vi "OldUWBController.vi"() -> ()   [LabVIEW 2016]
doc: "The roboRIO Project template acquires acceleration data from the onboard accelerometer and displays the changes of acceleration values in a waveform chart."
uses:
  <vilib>/myRIO/Instrument Drivers/Onboard IO/UART/typedef/VISA Configuration.ctl
  <vilib>/myRIO/Instrument Drivers/Onboard IO/UART/UART.lvlib
  <vilib>/Instr/_visa.llb/VISA Configure Serial Port (Instr).vi
  <vilib>/regexp/Match Regular Expression.xnode
  <vilib>/myRIO/Express VI/Onboard IO/UART/UART Express VI.xnode
panel:
  out "Character Count":u32
  out "UART Reset Buffer":string
  in  "Reset Active\n(Default: ON)":bool
  in  "Delay Time (s)":dbl=10.0
  in  "Stop Program":bool
  out "Z":dbl
  out "Y":dbl
  out "X":dbl
  out "offset past match\n(-1 = no match)":i32
  out "after POS match":string
  out "Characters Read":string
  out "error out OUTPUT":errorcluster
  in  "error in OUTPUT":errorcluster
  out "error out INPUT":errorcluster
  in  "error in INPUT":errorcluster
  # "UART INIT INPUT"
  # "UART OUTPUT"
  # "DEBUG"
  # "COORDINATES"
  # "Input ASCII Codes\n--------------------\nlep - 108, 101, 112\nlec - 108, 101, 99\n\ncr - 13"
  # "STARTUP RESET"
  # "INPUT ERROR"
  # "OUTPUT ERROR"
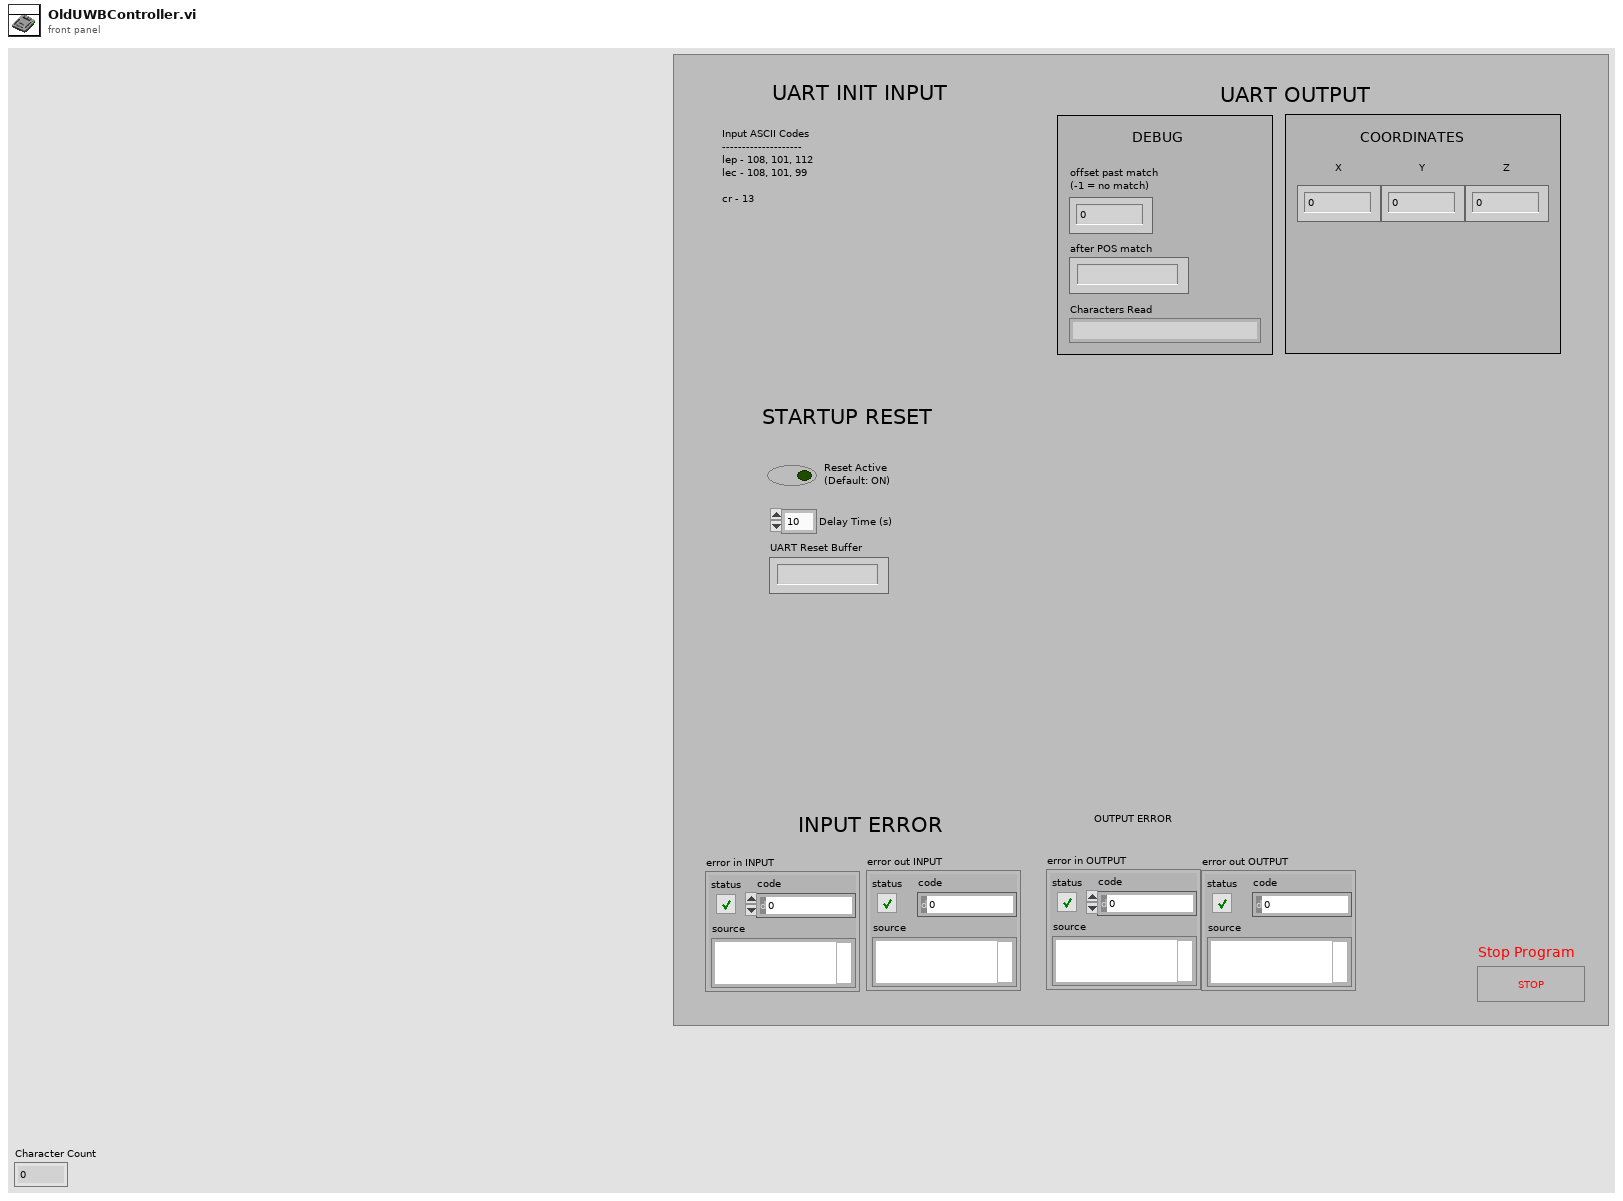
[diagram p1: front panel]
types:
  T1 = typedef "UART.lvlib/VISA Configuration.ctl" = cluster{"baud rate (9600)":u32, "data bits (8)":u16, "parity (0:none)":enum16{"None", "Odd", "Even", "Mark", "Space"}, "stop bits (10: 1 bit)":u16, "flow control (0:none)":u16, "termination char\n(0xA = '\\n' = LF) ":u8, "Enable Termination\nChar (T)":bool, "timeout (10sec)":u32}
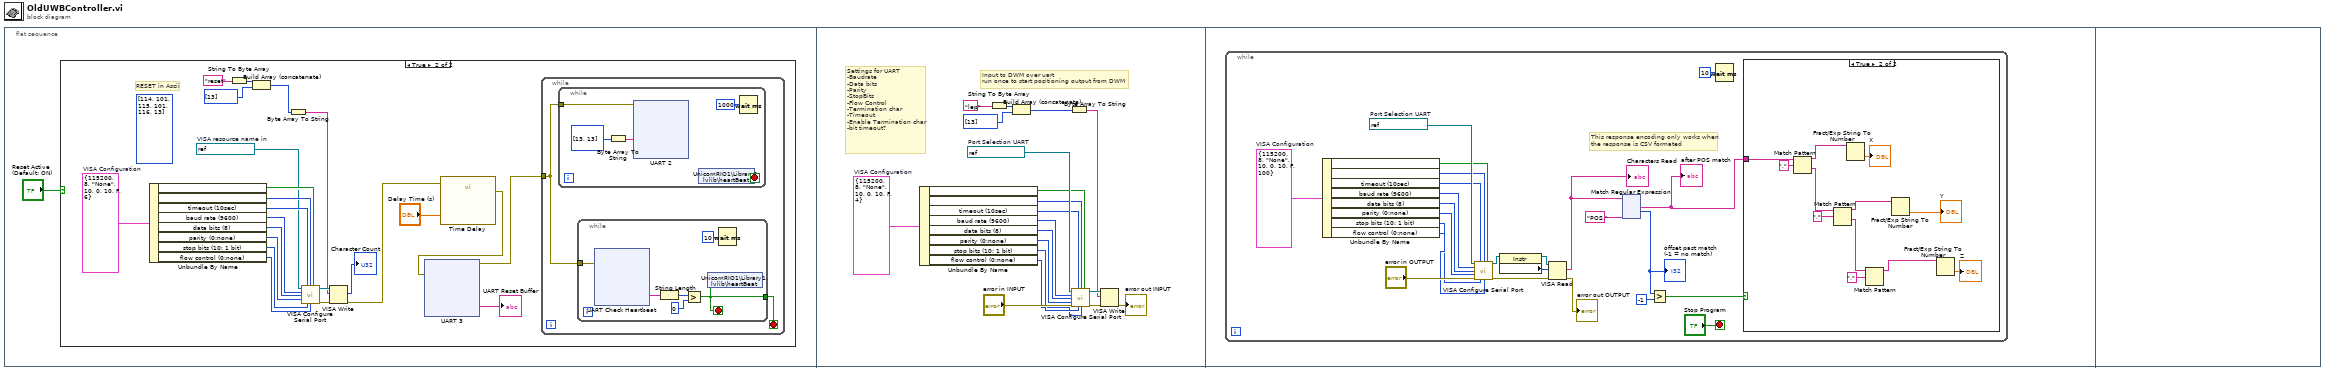
[diagram p0: block diagram]
diagram:
  n1 = flat-sequence {
    frame #0 {
      n2 = case shown="True" "Reset Active\n(Default: ON)" {
        frame False {
        }
        frame True {
          (unwired) u8[] [114, 101, 115, 101, 116, 13] ("unsigned byte array")
          w9 = T1 {"baud rate (9600)"=115200, "data bits (8)"=8, "parity (0:none)"=enum."None", "stop bits (10: 1 bit)"=10, "flow control (0:none)"=0, "termination char\n(0xA = '\\n' = LF) "=10, "Enable Termination\nChar (T)"=FALSE, "timeout (10sec)"=6}  # VISA Configuration
          w8 = refnum<visa-resource-name> "ASRL2::INSTR"  # VISA resource name in
          # "RESET in Ascii"
          n3 = Unbundle By Name(w9) -> ("Enable Termination\nChar (T)"=w13:bool, "termination char\n(0xA = '\\n' = LF)"=w14:u8, "timeout (10sec)"=w15:u32, "baud rate (9600)"=w20:u32, "data bits (8)"=w19:u16, "parity (0:none)"=w18:enum16{"None", "Odd", "Even", "Mark", "Space"}, "stop bits (10: 1 bit)"=w17:u16, "flow control (0:none)"=w16:u16)
          n4 = String To Byte Array(string="reset") -> (unsigned byte array=w4:u8[])
          n5 = Build Array (concatenate)(w4, i32[] [13]) -> (w3:i32[])
          n6 = Byte Array To String(unsigned byte array=w3) -> (string=w2:string)
          n7 = call-poly "VISA Configure Serial Port"("VISA resource name"=w8, "timeout (10sec)"=w15, "termination char\n(0xA = '\\n' = LF)"=w14, "Enable Termination\nChar (T)"=w13, "baud rate (9600)"=w20, "data bits (8)"=w19, "parity (0:none)"=w18, "stop bits (10: 1 bit)"=w17, "flow control (0:none)"=w16) -> ("VISA resource name out"=w11:refnum<visa-resource-name>, "error out"=w12:errorcluster)  [unwired: 5 in]
          n8 = VISA Write(VISA resource name=w11, write buffer=w2, error in (no error)=w12) -> (return count=→"Character Count":u32, error out=w7:errorcluster)  [unwired: 1 out]
          n9 = call "Time Delay"("error in (no error)"=w7, "Delay Time (s)"="Delay Time (s)") -> ("error out"=w22:errorcluster)  [unwired: 9 in]
          n10 = xnode "UART 3"("error in (no error)"=w22) -> ("Characters Read"=→"UART Reset Buffer":string, "error out"=w21:errorcluster)
          n11 = while {
            tunnel: w21 -> [w43]
            stop <- w42 stop-if-true
            n12 = while {
              tunnel: w43 -> [w45]
              stop <- w44 stop-if-true
              n13 = Byte Array To String(unsigned byte array=u8[] [13, 13]) -> (string=w48:string)
              n14 = xnode "UART 2"("Characters to Write"=w48, "error in (no error)"=w45) -> ()  [unwired: 2 out]
              n15 = shared-variable "UnicornRIO1\\Library1.lvlib\\heartBeat"() -> (w44:bool)  [unwired: 1 in, 1 out]
              n16 = Wait (ms)(milliseconds to wait=u32 1000) -> ()  [unwired: 1 out]
            }
            n17 = while {
              tunnel: [w65] -> w42
              tunnel: w43 -> [w66]
              stop <- w65 stop-if-true
              n18 = xnode "UART Check Heartbeat"("error in (no error)"=w66) -> ("Characters Read"=w70:string)  [unwired: 1 out]
              n19 = String Length(string=w70) -> (length=w69:i32)
              n20 = Greater?(x=w69, y=0) -> (0:w65:bool)
              n21 = shared-variable "UnicornRIO1\\Library1.lvlib\\heartBeat"(w65) -> ()  [unwired: 1 in, 1 out]
              n22 = Wait (ms)(milliseconds to wait=u32 10) -> ()  [unwired: 1 out]
            }
          }
        }
      }
    }
    frame #1 {
      w105 = T1 {"baud rate (9600)"=115200, "data bits (8)"=8, "parity (0:none)"=enum."None", "stop bits (10: 1 bit)"=10, "flow control (0:none)"=0, "termination char\n(0xA = '\\n' = LF) "=10, "Enable Termination\nChar (T)"=FALSE, "timeout (10sec)"=4}  # VISA Configuration
      w106 = refnum<visa-resource-name> "ASRL2::INSTR"  # Port Selection UART
      # "Input to DWM over uart\nrun once to start positioning output from DWM"
      # "Settings for UART\n-Baudrate\n-Data bits\n-Parity\n-StopBits\n-Flow Control\n-Termination char\n-Timeout\n-Enable Termination char\n-bit timeout?"
      n23 = Unbundle By Name(w105) -> ("Enable Termination\nChar (T)"=w100:bool, "termination char\n(0xA = '\\n' = LF)"=w99:u8, "timeout (10sec)"=w98:u32, "baud rate (9600)"=w94:u32, "data bits (8)"=w95:u16, "parity (0:none)"=w96:enum16{"None", "Odd", "Even", "Mark", "Space"}, "stop bits (10: 1 bit)"=w97:u16, "flow control (0:none)"=w92:u16)
      n24 = String To Byte Array(string="lep") -> (unsigned byte array=w89:u8[])
      n25 = Build Array (concatenate)(w89, i32[] [13]) -> (w88:i32[])
      n26 = Byte Array To String(unsigned byte array=w88) -> (string=w93:string)
      n27 = call-poly "VISA Configure Serial Port"("VISA resource name"=w106, "timeout (10sec)"=w98, "termination char\n(0xA = '\\n' = LF)"=w99, "Enable Termination\nChar (T)"=w100, "baud rate (9600)"=w94, "data bits (8)"=w95, "parity (0:none)"=w96, "error in (no error)"="error in INPUT", "stop bits (10: 1 bit)"=w97, "flow control (0:none)"=w92) -> ("VISA resource name out"=w103:refnum<visa-resource-name>, "error out"=w102:errorcluster)  [unwired: 4 in]
      n28 = VISA Write(VISA resource name=w103, write buffer=w93, error in (no error)=w102) -> (error out=→"error out INPUT":errorcluster)  [unwired: 2 out]
    }
    frame #2 {
      n29 = while {
        stop <- "Stop Program" stop-if-true
        w129 = T1 {"baud rate (9600)"=115200, "data bits (8)"=8, "parity (0:none)"=enum."None", "stop bits (10: 1 bit)"=10, "flow control (0:none)"=0, "termination char\n(0xA = '\\n' = LF) "=10, "Enable Termination\nChar (T)"=FALSE, "timeout (10sec)"=100}  # VISA Configuration
        w130 = refnum<visa-resource-name> "ASRL2::INSTR"  # Port Selection UART
        # "This response encoding only works when\nthe response is CSV formated"
        n30 = Unbundle By Name(w129) -> ("Enable Termination\nChar (T)"=w124:bool, "termination char\n(0xA = '\\n' = LF)"=w123:u8, "timeout (10sec)"=w122:u32, "baud rate (9600)"=w117:u32, "data bits (8)"=w118:u16, "parity (0:none)"=w119:enum16{"None", "Odd", "Even", "Mark", "Space"}, "stop bits (10: 1 bit)"=w120:u16, "flow control (0:none)"=w121:u16)
        n31 = call-poly "VISA Configure Serial Port"("VISA resource name"=w130, "timeout (10sec)"=w122, "termination char\n(0xA = '\\n' = LF)"=w123, "Enable Termination\nChar (T)"=w124, "baud rate (9600)"=w117, "data bits (8)"=w118, "parity (0:none)"=w119, "error in (no error)"="error in OUTPUT", "stop bits (10: 1 bit)"=w120, "flow control (0:none)"=w121) -> ("VISA resource name out"=w127:refnum<visa-resource-name>, "error out"=w126:errorcluster)  [unwired: 4 in]
        n32 = property class="Instr"(reference=w127) -> (reference out=w115:refnum<visa-resource-name>, "Serial Settings:Number of Bytes at Serial Port"=w116:u32)  [unwired: 1 in, 1 out]
        n33 = VISA Read(VISA resource name=w115, byte count=w116, error in (no error)=w126) -> (read buffer=w110:string, error out=→"error out OUTPUT":errorcluster)  [unwired: 2 out]
        "Characters Read" <- w110
        n34 = xnode "Match Regular Expression"("input string"=w110, "regular expression"="POS,") -> ("after match"=w109:string, "offset past match"=w112:i32)  [unwired: 4 in, 3 out]
        "after POS match" <- w109
        "offset past match\n(-1 = no match)" <- w112
        n35 = Greater?(x=w112, y=-1) -> (0:w108:bool)
        n36 = Wait (ms)(milliseconds to wait=u32 10) -> ()  [unwired: 1 out]
        n37 = case shown="True" w108 {
          tunnel: w109 -> [_ w131]
          frame False {
          }
          frame True {
            n38 = Match Pattern(string=w131, regular expression=",") -> (before substring=w141:string, after substring=w137:string)  [unwired: 1 in, 2 out]
            n39 = Match Pattern(string=w137, regular expression=",") -> (before substring=w135:string, after substring=w136:string)  [unwired: 1 in, 2 out]
            n40 = Fract/Exp String To Number(string=w141) -> (number=→"X":dbl)  [unwired: 3 in, 1 out]
            n41 = Match Pattern(string=w136, regular expression=",") -> (before substring=w134:string)  [unwired: 1 in, 3 out]
            n42 = Fract/Exp String To Number(string=w135) -> (number=→"Y":dbl)  [unwired: 3 in, 1 out]
            n43 = Fract/Exp String To Number(string=w134) -> (number=→"Z":dbl)  [unwired: 3 in, 1 out]
          }
        }
      }
    }
    frame #3 {
    }
  }
